vi "ELVIS III v1.1 Open DO (N Samples).vi"(7 "Allow multiple opens?":bool, 8 "error in (no error)":errorcluster, 10 "Channel Names":string[](array[string]), 11 "Resource name":T3 caption="RIO Device") -> (0 "error out":errorcluster, 2 "DO (N Samples) Channel List":T4, 3 "myRIO Ref Out":T1)   [LabVIEW 2021]
uses:
  <vilib>/myRIO/Common/Instrument Driver Framework/myRIO v1.0/DO Block/typedefs/DO Block Channels List.ctl
  <vilib>/myRIO/Common/Instrument Driver Framework/myRIO v1.0/DO Block/typedefs/DO Block Channels Enum.ctl
  <vilib>/userDefined/High Color/nirio_resource_hc.ctl
  <vilib>/myRIO/Common/Instrument Driver Framework/Utilities/typedefs/myRIO v1.0 Reference.ctl
  <vilib>/myRIO/Common/Instrument Driver Framework/Utilities/typedefs/Generic FPGA Reference.ctl
  <vilib>/myRIO/Common/Instrument Driver Framework/ELVIS III v1.0/DO Block/typedefs/ELVIS III v1.0 DO Block Channels Enum.ctl
  <vilib>/Utility/VariantDataType/GetNumericInfo.vi
  <vilib>/Utility/error.llb/Error Cluster From Error Code.vi
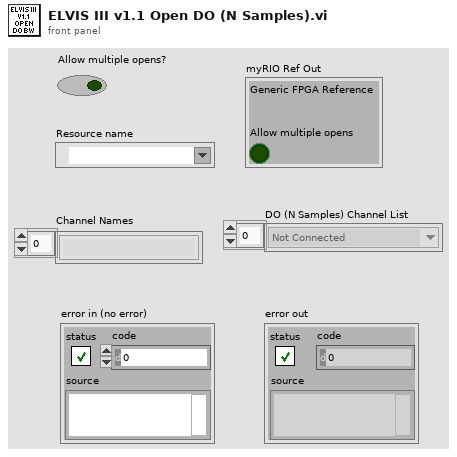
[diagram p1: front panel]
types:
  T1 = typedef "myRIO v1.0 Reference.ctl" = cluster{"Generic FPGA Reference":T2, "Allow multiple opens":bool}
  T2 = typedef "Generic FPGA Reference.ctl" = refnum<k20>
  T3 = typedef "nirio_resource_hc.ctl" = tag
  T4 = typedef "DO Block Channels List.ctl" = T5[]
  T5 = typedef "DO Block Channels Enum.ctl" = enum16{"Not Connected", "A/DO0 (N Samples)", "A/DO1 (N Samples)", "A/DO2 (N Samples)", "A/DO3 (N Samples)", "A/DO4 (N Samples)", "A/DO5 (N Samples)", "A/DO6 (N Samples)", "A/DO7 (N Samples)", "A/DO8 (N Samples)", "A/DO9 (N Samples)", "A/DO10 (N Samples)", "A/DO11 (N Samples)", "A/DO12 (N Samples)", "A/DO13 (N Samples)", "A/DO14 (N Samples)", "A/DO15 (N Samples)", "A/DO16 (N Samples)", "A/DO17 (N Samples)", "A/DO18 (N Samples)", "A/DO19 (N Samples)", "B/DO0 (N Samples)", "B/DO1 (N Samples)", "B/DO2 (N Samples)", "B/DO3 (N Samples)", "B/DO4 (N Samples)", "B/DO5 (N Samples)", "B/DO6 (N Samples)", "B/DO7 (N Samples)", "B/DO8 (N Samples)", "B/DO9 (N Samples)", "B/DO10 (N Samples)", "B/DO11 (N Samples)", "B/DO12 (N Samples)", "B/DO13 (N Samples)", "B/DO14 (N Samples)", "B/DO15 (N Samples)", "B/DO16 (N Samples)", "B/DO17 (N Samples)", "B/DO18 (N Samples)", "B/DO19 (N Samples)"}
  T6 = typedef "ELVIS III v1.0 DO Block Channels Enum.ctl" = enum16{"Not Connected", "A/DO0 (N Samples)", "A/DO1 (N Samples)", "A/DO2 (N Samples)", "A/DO3 (N Samples)", "A/DO4 (N Samples)", "A/DO5 (N Samples)", "A/DO6 (N Samples)", "A/DO7 (N Samples)", "A/DO8 (N Samples)", "A/DO9 (N Samples)", "A/DO10 (N Samples)", "A/DO11 (N Samples)", "A/DO12 (N Samples)", "A/DO13 (N Samples)", "A/DO14 (N Samples)", "A/DO15 (N Samples)", "A/DO16 (N Samples)", "A/DO17 (N Samples)", "A/DO18 (N Samples)", "A/DO19 (N Samples)", "B/DO0 (N Samples)", "B/DO1 (N Samples)", "B/DO2 (N Samples)", "B/DO3 (N Samples)", "B/DO4 (N Samples)", "B/DO5 (N Samples)", "B/DO6 (N Samples)", "B/DO7 (N Samples)", "B/DO8 (N Samples)", "B/DO9 (N Samples)", "B/DO10 (N Samples)", "B/DO11 (N Samples)", "B/DO12 (N Samples)", "B/DO13 (N Samples)", "B/DO14 (N Samples)", "B/DO15 (N Samples)", "B/DO16 (N Samples)", "B/DO17 (N Samples)", "B/DO18 (N Samples)", "B/DO19 (N Samples)"}
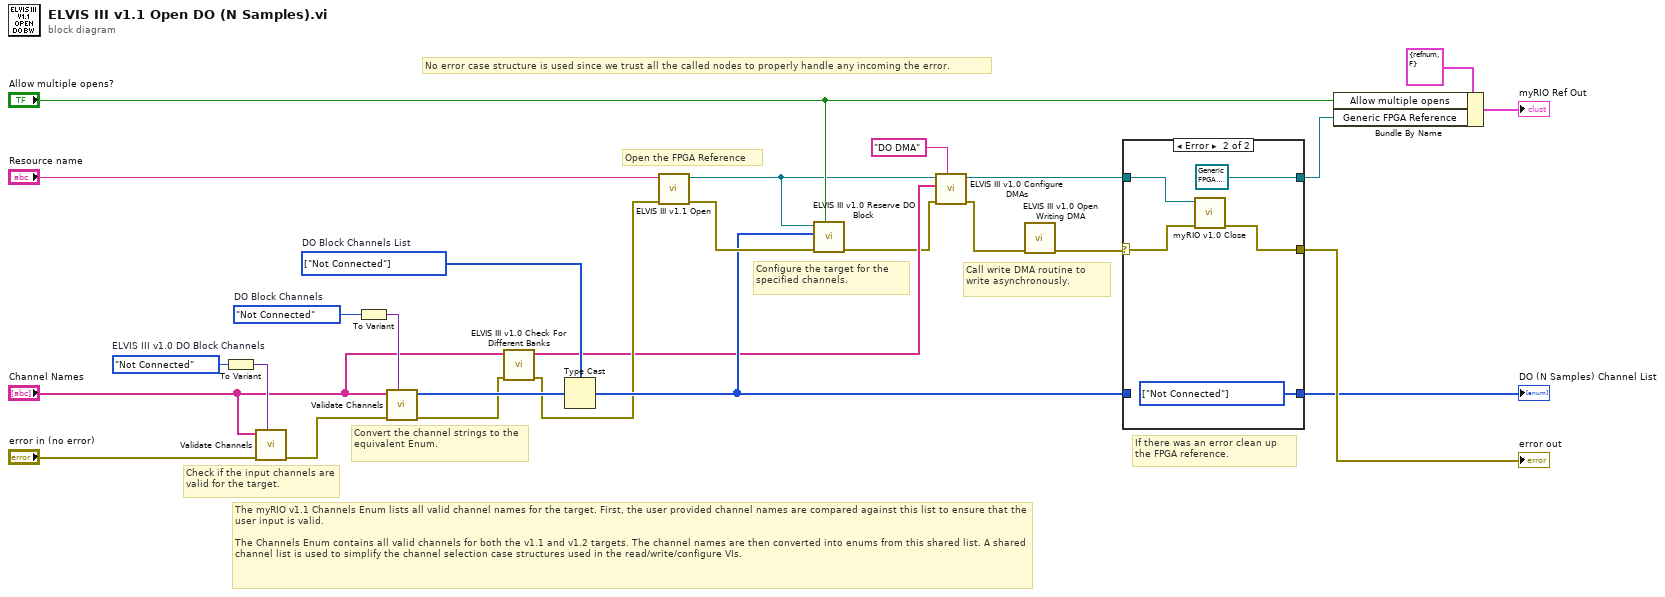
[diagram p0: block diagram]
diagram:
  w13 = T4 [enum."Not Connected"] items=["Not Connected", "A/DO0 (N Samples)", "A/DO1 (N Samples)", "A/DO2 (N Samples)", "A/DO3 (N Samples)", "A/DO4 (N Samples)", "A/DO5 (N Samples)", "A/DO6 (N Samples)", "A/DO7 (N Samples)", "A/DO8 (N Samples)", "A/DO9 (N Samples)", "A/DO10 (N Samples)", "A/DO11 (N Samples)", "A/DO12 (N Samples)", "A/DO13 (N Samples)", "A/DO14 (N Samples)", "A/DO15 (N Samples)", "A/DO16 (N Samples)", "A/DO17 (N Samples)", "A/DO18 (N Samples)", "A/DO19 (N Samples)", "B/DO0 (N Samples)", "B/DO1 (N Samples)", "B/DO2 (N Samples)", "B/DO3 (N Samples)", "B/DO4 (N Samples)", "B/DO5 (N Samples)", "B/DO6 (N Samples)", "B/DO7 (N Samples)", "B/DO8 (N Samples)", "B/DO9 (N Samples)", "B/DO10 (N Samples)", "B/DO11 (N Samples)", "B/DO12 (N Samples)", "B/DO13 (N Samples)", "B/DO14 (N Samples)", "B/DO15 (N Samples)", "B/DO16 (N Samples)", "B/DO17 (N Samples)", "B/DO18 (N Samples)", "B/DO19 (N Samples)"]  # DO Block Channels List
  w14 = DO_Block_Channels_Enum."Not Connected"  # DO Block Channels
  w15 = ELVIS_III_v1.0_DO_Block_Channels_Enum."Not Connected"  # ELVIS III v1.0 DO Block Channels
  # "Call write DMA routine to write asynchronously."
  # "The myRIO v1.1 Channels Enum lists all valid channel names for the target. First, the user provided channel names are compared against this list to ensure that the user input is valid.\n\nThe Channels Enum contains all valid channels for both the v1.1 and v1.2 targets. The channel names are then converted into enums from this shared list. A shared channel list is used to simplify the channel selection case structures used in the read/write/configure VIs."
  # "If there was an error clean up the FPGA reference."
  # "Configure the target for the specified channels."
  # "Open the FPGA Reference"
  # "No error case structure is used since we trust all the called nodes to properly handle any incoming the error."
  # "Convert the channel strings to the equivalent Enum."
  # "Check if the input channels are valid for the target."
  n1 = To Variant(anything=w15) -> (Variant=w16:variant)
  n2 = call <vilib>:"Validate Channels.vi"("Channels Enum Variant"=w16, "error in (no error)"="error in (no error)", "Channel Names"="Channel Names") -> ("error out"=w25:errorcluster)  [unwired: 7 in, 1 out]
  n3 = To Variant(anything=w14) -> (Variant=w17:variant)
  n4 = call <vilib>:"Validate Channels.vi"("Channels Enum Variant"=w17, "error in (no error)"=w25, "Channel Names"="Channel Names") -> ("error out"=w8:errorcluster, "Index Array"=w22:u16[])  [unwired: 7 in]
  n5 = call <vilib>:"ELVIS III v1.0 Check For Different Banks.vi"("error in (no error)"=w8, "Channel Names"="Channel Names") -> ("error out"=w7:errorcluster)  [unwired: 9 in]
  n6 = Type Cast(type=w13, x=w22) -> (*(type *) &x=w9:T4)
  n7 = call <vilib>:"ELVIS III v1.1 Open.vi"("error in (no error)"=w7, "Resource name"="Resource name") -> ("error out"=w21:errorcluster, "myRIO FPGA Ref Out"=w6:T2)  [unwired: 8 in]
  n8 = call <vilib>:"ELVIS III v1.0 Reserve DO Block.vi"("Allow multiple opens?"="Allow multiple opens?", "error in (no error)"=w21, "DO (N Samples) Channel List"=w9, "Generic FPGA Reference"=w6) -> ("error out"=w3:errorcluster)  [unwired: 7 in]
  n9 = call <vilib>:"ELVIS III v1.0 Configure DMAs.vi"("DMA Type"="DO DMA", "error in (no error)"=w3, "Channel Names"="Channel Names", "ELVIS III FPGA Ref"=w6) -> ("error out"=w2:errorcluster, "ELVIS III FPGA Ref"=w5:T2)  [unwired: 6 in]
  n10 = call <vilib>:"ELVIS III v1.0 Open Writing DMA.vi"("error in (no error)"=w2) -> ("error out"=w10:errorcluster)  [unwired: 10 in]
  n11 = case shown="Error" w10 {
    selector: w10 -> [w28 w34]
    tunnel: w5 -> [w29 w32]
    tunnel: [w29 T2 refnum ("myRIO FPGA Ref Out")] -> w18
    tunnel: [w28 w33] -> w23
    tunnel: w9 -> [w27 _]
    tunnel: [w27 w30] -> w20
    frame No Error {
    }
    frame Error {
      w30 = T4 [enum."Not Connected"] items=["Not Connected", "A/DO0 (N Samples)", "A/DO1 (N Samples)", "A/DO2 (N Samples)", "A/DO3 (N Samples)", "A/DO4 (N Samples)", "A/DO5 (N Samples)", "A/DO6 (N Samples)", "A/DO7 (N Samples)", "A/DO8 (N Samples)", "A/DO9 (N Samples)", "A/DO10 (N Samples)", "A/DO11 (N Samples)", "A/DO12 (N Samples)", "A/DO13 (N Samples)", "A/DO14 (N Samples)", "A/DO15 (N Samples)", "A/DO16 (N Samples)", "A/DO17 (N Samples)", "A/DO18 (N Samples)", "A/DO19 (N Samples)", "B/DO0 (N Samples)", "B/DO1 (N Samples)", "B/DO2 (N Samples)", "B/DO3 (N Samples)", "B/DO4 (N Samples)", "B/DO5 (N Samples)", "B/DO6 (N Samples)", "B/DO7 (N Samples)", "B/DO8 (N Samples)", "B/DO9 (N Samples)", "B/DO10 (N Samples)", "B/DO11 (N Samples)", "B/DO12 (N Samples)", "B/DO13 (N Samples)", "B/DO14 (N Samples)", "B/DO15 (N Samples)", "B/DO16 (N Samples)", "B/DO17 (N Samples)", "B/DO18 (N Samples)", "B/DO19 (N Samples)"] ("DO Block Write Channels List")
      n12 = call <vilib>:"myRIO v1.0 Close.vi"("error in (no error)"=w34, "myRIO FPGA Ref In"=w32) -> ("error out"=w33:errorcluster)  [unwired: 9 in]
    }
  }
  "DO (N Samples) Channel List" <- w20
  "error out" <- w23
  n13 = Bundle By Name(cluster=T1 {"Generic FPGA Reference"=refnum, "Allow multiple opens"=FALSE} ("myRIO Ref Out"), "Allow multiple opens"="Allow multiple opens?", "Generic FPGA Reference"=w18) -> (→"myRIO Ref Out":T1)
